vi "Get Variant Message.vi"(8 "error in (no error)":errorcluster, 11 "Message Response in":refnum<class "Message Response.lvclass">) -> (0 "error out":errorcluster, 1 "Value":variant, 2 "Name":string, 3 "Message Response out":refnum<class "Message Response.lvclass">)   [LabVIEW 2016, in "WebSocket Networking.lvlib" / "Message Response.lvclass"]
doc: "--\nCopyright © 2017 Composed SystemsI All rights reserved.\n\nAuthor: Jon McBee <jon.mcbee@composed.io>\n\nThis library is provided \"AS IS\" ,WITHOUT WARRANTIES OR\nCONDITIONS OF ANY KIND, either express or implied.\n\nComposed Systems -- composed.io\n\nStream 0.0.1.1\nJon McBee - Composed Systems\nCopyright (c) 2017, Composed Systems"
uses:
  <userlib>/Common Components/WebSocket Networking/Message Response/Message Response.lvclass
  C:/Program Files (x86)/National Instruments/LabVIEW 2016/user.lib/Composed Systems/Stream/Mediator/Classes/Message Interface/Message Interface.lvclass
  <userlib>/Common Components/WebSocket Networking/Message Response/Message Response.lvclass/Message Response.ctl
  <userlib>/Composed Systems/Stream/Mediator/Classes/Message Interface/Get Name.vi
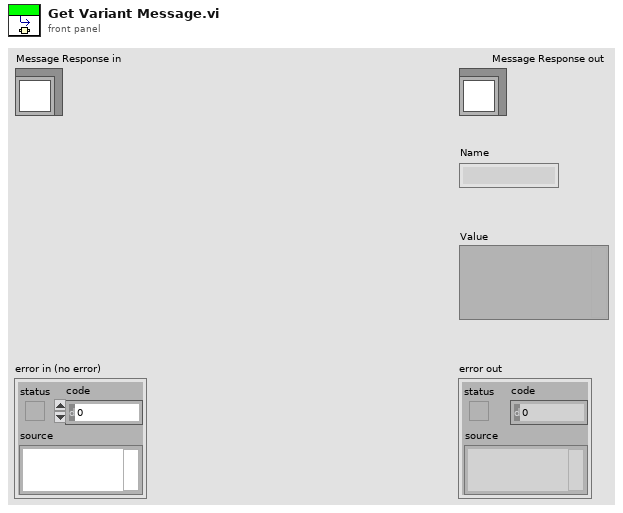
[diagram p1: front panel]
types:
  T1 = typedef "Common.lvlib/command-data.ctl" = cluster{"command":string, "data":string}
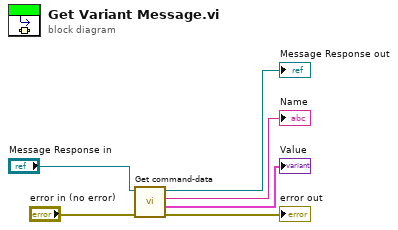
[diagram p0: block diagram]
diagram:
  n1 = call <userlib>:"Get command-data.vi"("error in (no error)"="error in (no error)", "Message Response in"="Message Response in") -> ("error out"=→"error out":errorcluster, "Cluster"=→"Value":T1, "Name"=→"Name":string, "Message Response out"=→"Message Response out":refnum<class "Message Response.lvclass">)  [unwired: 6 in]
